vi "Remote Controller.vi"() -> ()   [LabVIEW 2017]
uses:
  <vilib>/Skyline/Message/AMQP/sync/Open (Sync).vi
  <vilib>/Skyline/Tag/Wrapper/Wrapper AMQP_class/Query Tags AMQP.vi
  <vilib>/Skyline/Tag/Wrapper/Wrapper_class/Delete Tag (Multiple).vi
  <vilib>/Skyline/Tag/Wrapper/Wrapper_class/Close Tag (Multiple).vi
  <vilib>/Skyline/Message/AMQP/NI Skyline Message AMQP (Sync).lvclass
  <vilib>/Skyline/Tag/Wrapper/Wrapper_class/NI Skyline Tag.lvclass
  <vilib>/Skyline/Tag/Wrapper/Wrapper AMQP_class/NI Skyline Tag AMQP.lvclass
  <vilib>/Skyline/Message/NI Skyline Message.lvclass
panel:
  in  "delete":bool
  out "Total Tags":i32
  in  "query":bool
  in  "stop":bool
  out "Running":bool
  in  "start":bool
  in  "tag_updates":i32=1
  in  "tag_publish_interval":i32=1000
  in  "tag_count":i32=1
  in  "Exit":bool
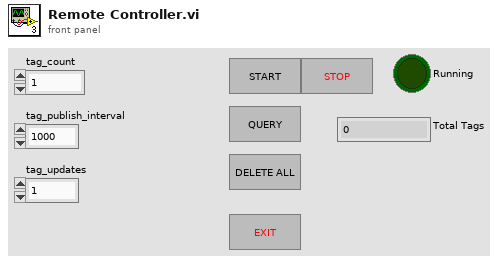
[diagram p1: front panel]
types:
  T1 = cluster{"tag_updates":i32, "tag_publish_interval":i32, "tag_count":i32}
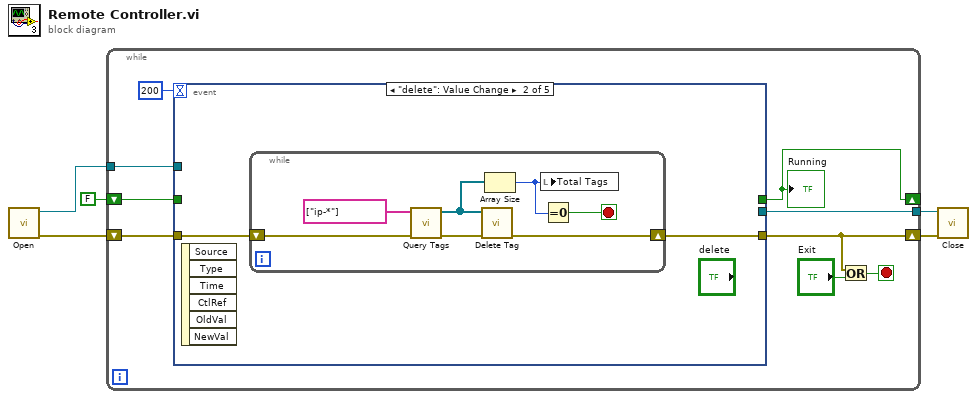
[diagram p0: block diagram]
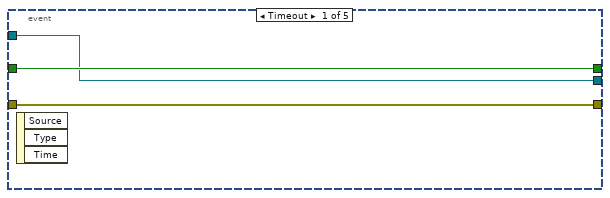
[diagram p2: hidden frame]
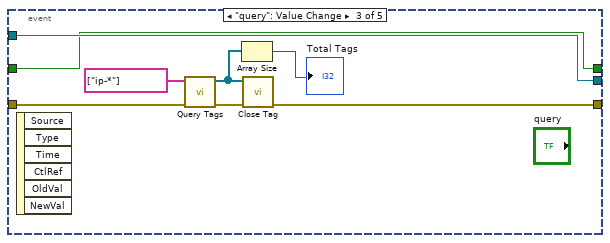
[diagram p3: hidden frame]
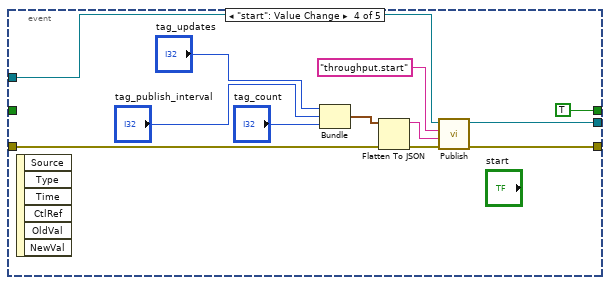
[diagram p4: hidden frame]
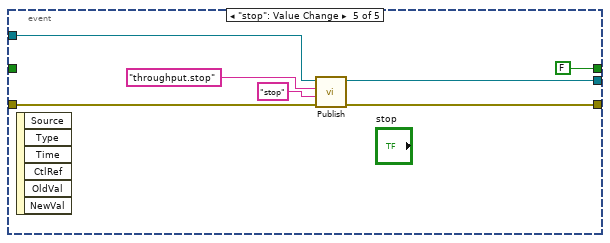
[diagram p5: hidden frame]
diagram:
  n1 = call-poly <vilib>:"Open.vi"() -> ("error out"=w3:errorcluster, "message sync out"=w4:refnum<class "NI Skyline Message AMQP (Sync).lvclass">)  [unwired: 10 in]
  n2 = while {
    shift-right: [w13] -> _
    shift-left: FALSE ("start") -> [w12]
    tunnel: w4 -> [w11]
    tunnel: [w9] -> w2
    shift-right: [w8] -> w1
    shift-left: w3 -> [w10]
    stop <- w7 stop-if-true
    n3 = event shown="[1] \"delete\": Value Change" {
      selector: _ -> [_ _ _ _ _]
      dyn-events: _ -> [_ _ _ _ _]
      timeout: 200 -> [_ _ _ _ _]
      tunnel: [w17 _ w28 TRUE ("start") FALSE ("start")] -> w13
      tunnel: w12 -> [w17 _ w28 _ _]
      tunnel: w11 -> [w16 _ w34 w45 w53]
      tunnel: w10 -> [w15 w19 w33 w39 w52]
      tunnel: [w16 _ w34 w43 w49] -> w9
      tunnel: [w15 w18 w30 w44 w48] -> w8
      event Timeout {
        n4 = event-data() -> ()  [unwired: 1 in, 3 out]
      }
      event "delete": Value Change {
        n5 = event-data() -> ()  [unwired: 1 in, 6 out]
        n6 = while {
          shift-right: [w24] -> w18
          shift-left: w19 -> [w26]
          stop <- w20 stop-if-true
          n7 = call-poly <vilib>:"Query Tags.vi"("error in (no error)"=w26, "paths (*)"=string[] ["ip-*"]) -> ("error out"=w25:errorcluster, "tags"=w23:refnum<class "NI Skyline Tag.lvclass">[])  [unwired: 8 in]
          n8 = call-poly <vilib>:"Delete Tag.vi"("error in (no error)"=w25, "tags in"=w23) -> ("error out"=w24:errorcluster)  [unwired: 9 in]
          n9 = Array Size(array=w23) -> (size(s)=w21:i32)
          n10 = local write "Total Tags"(w21) -> ()
          n11 = Equal To 0?(x=w21) -> (x = 0?=w20:bool)
        }
      }
      event "query": Value Change {
        n12 = event-data() -> ()  [unwired: 1 in, 6 out]
        n13 = call-poly <vilib>:"Query Tags.vi"("error in (no error)"=w33, "paths (*)"=string[] ["ip-*"]) -> ("error out"=w31:errorcluster, "tags"=w32:refnum<class "NI Skyline Tag.lvclass">[])  [unwired: 8 in]
        n14 = Array Size(array=w32) -> (size(s)=→"Total Tags":i32)
        n15 = call-poly <vilib>:"Close Tag.vi"("error in (no error)"=w31, "tags in"=w32) -> ("error out"=w30:errorcluster)  [unwired: 9 in]
      }
      event "start": Value Change {
        n16 = event-data() -> ()  [unwired: 1 in, 6 out]
        n17 = Bundle("tag_updates"="tag_updates", "tag_publish_interval"="tag_publish_interval", "tag_count"="tag_count") -> (w36:T1)  [unwired: 1 in]
        n18 = Flatten To JSON(anything=w36, error in (no error)=w39) -> (JSON string=w41:string, 11:w40:errorcluster)  [unwired: 1 in]
        n19 = call-dynamic "Publish.vi"("error in (no error)"=w40, "message"=w41, "topic"="throughput.start", "message sync"=w45) -> ("error out"=w44:errorcluster, "message sync out"=w43:refnum<class "NI Skyline Message AMQP (Sync).lvclass">)  [unwired: 6 in]
      }
      event "stop": Value Change {
        n20 = event-data() -> ()  [unwired: 1 in, 6 out]
        n21 = call-dynamic "Publish.vi"("error in (no error)"=w52, "message"="stop", "topic"="throughput.stop", "message sync"=w53) -> ("error out"=w48:errorcluster, "message sync out"=w49:refnum<class "NI Skyline Message AMQP (Sync).lvclass">)  [unwired: 6 in]
      }
    }
    "Running" <- w13
    n22 = Or(x=w8, y="Exit") -> (x .or. y?=w7:bool)
  }
  n23 = call-dynamic "Close.vi"("error in (no error)"=w1, "message sync"=w2) -> ()  [unwired: 9 in, 1 out]
